vi "Init.vi"(8 "error in (no error)":errorcluster, 11 "uService Template in":refnum<class "Template Internal uService.lvclass">) -> (0 "error out":errorcluster, 3 "uService Template out":refnum<class "Template Internal uService.lvclass">)   [LabVIEW 2026, in "TALOS.lvlib" / "Template Internal uService.lvlib" / "Template Internal uService.lvclass"]
uses:
  Template Internal uService.lvclass
  C:/LabVIEW Code/TALOS/talos/Ancestor/Ancestor/Ancestor.lvclass
  C:/LabVIEW Code/TALOS/talos/Father of all uServices/Father of all uServices/Father of all uServices.lvclass
  Ancestor/Ancestor/Ancestor.lvclass/Ancestor.ctl
  Father of all uServices/Father of all uServices/Father of all uServices.lvclass/Father of all uServices.ctl
  Support VIs/Substitute Error.vi
  Support VIs/Generate Error.vi
  FGV/Error Memory/Get Error Description.vi
  Support VIs/Get PC name.vi
  Support VIs/Get Class Name.vi
  <vilib>/Utility/error.llb/Clear Errors.vi
  FGV/Error Memory/Error Memory Core.vi
  <vilib>/AdvancedString/Delimited String to 1D String Array.vi
  <vilib>/AdvancedString/Delimited String to 1D String Array (string).vi
  Support VIs/Circus Root Path.vi
  FGV/Error Memory/Error Crt Lvl checker.vi
  FGV/Error Memory/Error Memory Core.vi/40c8088d-b597-4017-91af-faa98e00292e.vi
  FGV/Error Memory/Error Memory Core.vi/d4a3ab98-063c-4e44-b43d-fbdcfe6c2be2.vi
  Support VIs/Global Memory.vi
  <vilib>/Utility/LVClass/Get LV Class Name.vi
  Support VIs/Is in Packed Library.vi
  Support VIs/TALOS Root path.vi
  Support VIs/Read CSV worksheet.vi
  Support VIs/Global Constants.vi
  <vilib>/Utility/error.llb/General Error Handler.vi
  Support VIs/Error Log.vi
  Father of all uServices/Father of all uServices/Father of all uServices.lvclass
  Ancestor/Ancestor/Ancestor.lvclass
  <vilib>/Comparison/Equal/Equal Functor/Equal Functor.lvclass
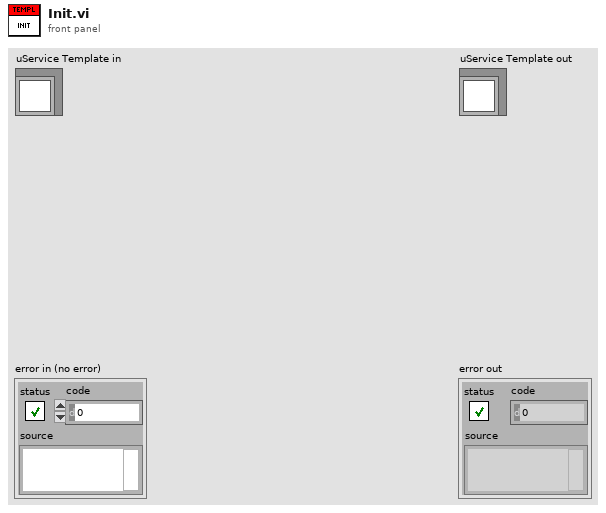
[diagram p1: front panel]
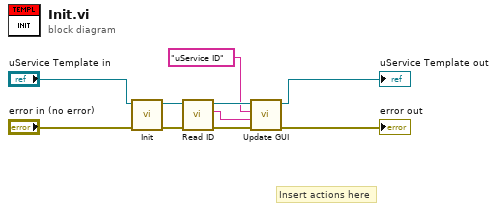
[diagram p0: block diagram]
diagram:
  # "Insert actions here"
  n1 = call-parent "Init.vi"("error in (no error)"="error in (no error)", "uService Template in"="uService Template in") -> ("error out"=w7:errorcluster, "uService Template out"=w8:refnum<class "Template Internal uService.lvclass">)  [unwired: 8 in]
  n2 = call "Read ID.vi"("error in (no error)"=w7, "Ancestor in"=w8) -> ("error out"=w6:errorcluster, "ID"=w3:string, "Ancestor out"=w5:refnum<class "Template Internal uService.lvclass">)  [unwired: 7 in]
  n3 = call "Update GUI.vi"("error in (no error)"=w6, "Data"=w3, "GUI Item Name"="uService ID", "uService Template in"=w5) -> ("error out"=→"error out":errorcluster, "uService Template out"=→"uService Template out":refnum<class "Template Internal uService.lvclass">)  [unwired: 6 in]
